vi "CalcState.vi"(8 "State":bool, 9 "Item":string, 10 "SwitchMap":T1(array[cluster]), 11 "States _n":bool[](array[boolean])) -> (3 "States_Out":bool[](array[boolean]))   [LabVIEW 2022 SP3, in "Switch_Manager.lvlib" / "Switch_Manager.lvclass"]
uses:
  Switch_Manager.lvclass
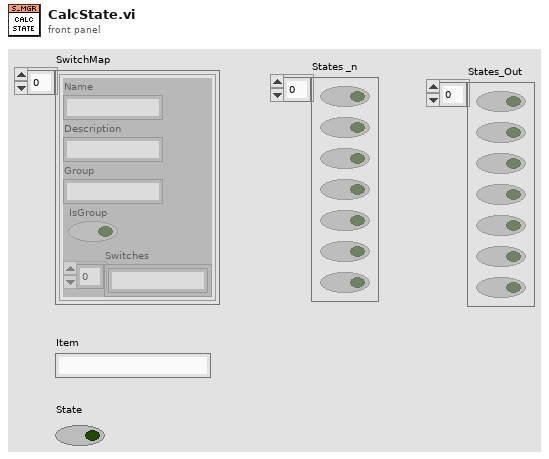
[diagram p1: front panel]
types:
  T1 = cluster{"Name":string, "Description":string, "Group":string, "IsGroup":bool, "Switches":string[]}[]
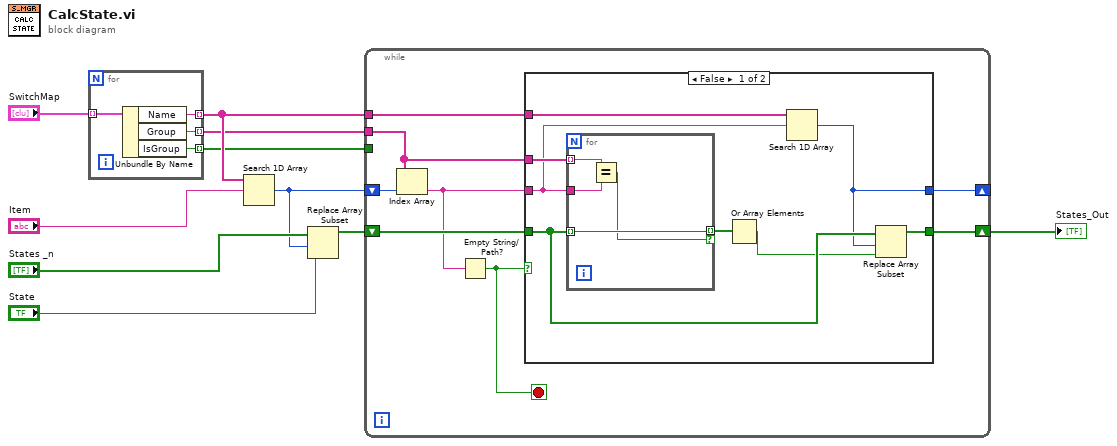
[diagram p0: block diagram]
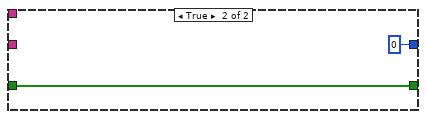
[diagram p2: hidden frame]
diagram:
  n1 = for {
    tunnel: "SwitchMap" -> [w14] mode=indexing
    tunnel: [w13] -> w7 mode=indexing
    tunnel: [w12] -> w6 mode=indexing
    tunnel: [w11] -> w5 mode=indexing
    n2 = Unbundle By Name(w14) -> ("Name"=w13:string, "Group"=w12:string, "IsGroup"=w11:bool)
  }
  n3 = Search 1D Array(1D array=w7, element="Item") -> (index of element=w3:i32)  [unwired: 1 in]
  n4 = Replace Array Subset(array="States _n", new element="State", index=w3) -> (w8:bool[])
  n5 = while {
    shift-right: [w19] -> w2
    shift-left: w8 -> [w20]
    tunnel: w7 -> [w21]
    tunnel: w6 -> [w22]
    tunnel: w5 -> [_]
    shift-right: [w17] -> _
    shift-left: w3 -> [w18]
    stop <- w15 stop-if-true
    n6 = Index Array(array=w22, index=w18) -> (element=w16:string)
    n7 = Empty String/Path?(string/path=w16) -> (empty?=w15:bool)
    n8 = case shown="False" w15 {
      tunnel: w22 -> [w30 _]
      tunnel: w21 -> [w28 _]
      tunnel: w20 -> [w27 w36]
      tunnel: [w25 w36] -> w19
      tunnel: [w24 0 ("index of element")] -> w17
      tunnel: w16 -> [w23 _]
      frame False {
        n9 = for {
          tunnel: w27 -> [w32] mode=indexing
          tunnel: w23 -> [w33]
          tunnel: w30 -> [w34] mode=indexing
          tunnel: [w32] -> w29 mode=indexing if=w31
          n10 = Equal?(x=w34, y=w33) -> (x = y?=w31:bool)
        }
        n11 = Or Array Elements(Boolean array=w29) -> (logical OR=w26:bool)
        n12 = Search 1D Array(1D array=w28, element=w23) -> (index of element=w24:i32)  [unwired: 1 in]
        n13 = Replace Array Subset(array=w27, new element=w26, index=w24) -> (w25:bool[])
      }
      frame True {
      }
    }
  }
  "States_Out" <- w2
